vi "FirstVI.vi"() -> ()   [LabVIEW 2014]
panel:
  out "Kelvin":dbl
  out "Celsius":dbl
  in  "Farenheit":dbl
  out "Thermometer Farenheit":dbl(slide) scale=-148.0..212.0
  out "Thermometer Kelvin":dbl(slide) scale=173.0..373.0
  out "Thermometer Celsius":dbl(slide) scale=-100.0..100.0
  in  "x":dbl
  out "Tank":dbl(slide) scale=0.0..100.0
  in  "Dial":dbl(knob) scale=0.0..10.0
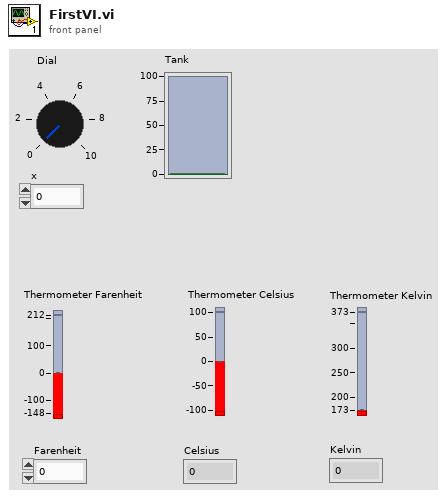
[diagram p1: front panel]
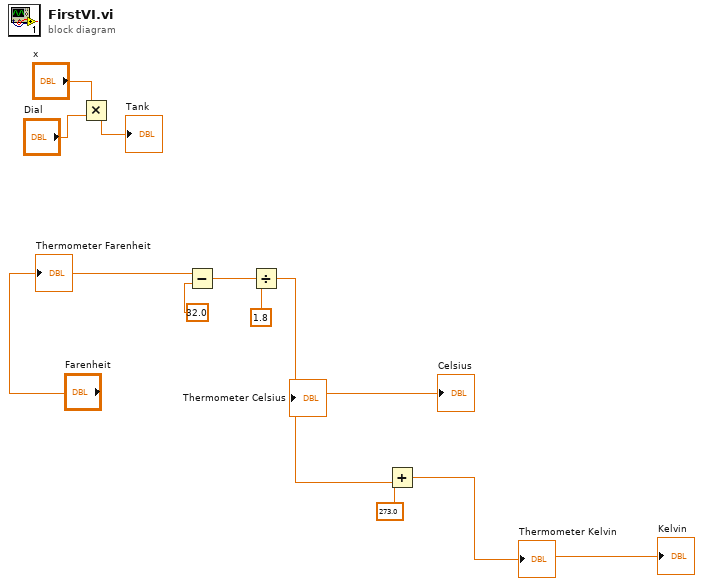
[diagram p0: block diagram]
diagram:
  n1 = Multiply(x="x", y="Dial") -> (x*y=→"Tank":dbl)
  n2 = Subtract(x="Farenheit", y=32.0) -> (x-y=w5:dbl)
  n3 = Divide(x=w5, y=1.8 ("x/y")) -> (x/y=w2:dbl)
  "Thermometer Celsius" <- w2
  "Celsius" <- w2
  n4 = Add(x=273.0, y=w2) -> (x+y=→"Thermometer Kelvin" →"Kelvin":dbl)
  "Thermometer Farenheit" <- "Farenheit"
